vi "Upd Range.vi"(8 "error in (no error)":errorcluster, 11 "FC2901 in":refnum<class "FC2901.lvclass">) -> (0 "error out":errorcluster, 3 "FC2901 out":refnum<class "FC2901.lvclass">)   [LabVIEW 2021, in "FC2901.lvclass"]
uses:
  FC2901.lvclass
  FC2901.lvclass/FC2901.ctl
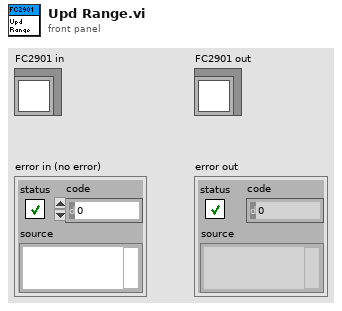
[diagram p1: front panel]
types:
  T1 = typedef "C100L.lvclass/GCF Data.ctl" = map{string, dbl}
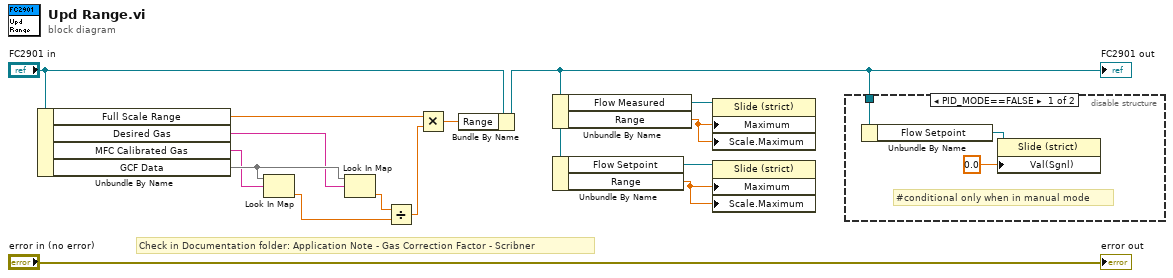
[diagram p0: block diagram]
diagram:
  # "Check in Documentation folder: Application Note - Gas Correction Factor - Scribner"
  n1 = Unbundle By Name("FC2901 in") -> ("Full Scale Range"=w10:dbl, "Desired Gas"=w11:string, "MFC Calibrated Gas"=w12:string, "GCF Data"=w13:T1)
  n2 = Look In Map(map=w13, key=w12) -> (value=w7:dbl)  [unwired: 1 in, 1 out]
  n3 = Look In Map(map=w13, key=w11) -> (value=w8:dbl)  [unwired: 1 in, 1 out]
  n4 = Divide(x=w8, y=w7) -> (x/y=w9:dbl)
  n5 = Multiply(x=w10, y=w9) -> (x*y=w2:dbl)
  n6 = Bundle By Name(cluster="FC2901 in", "Range"=w2) -> (w1:refnum<class "FC2901.lvclass">)
  "FC2901 out" <- w1
  n7 = Unbundle By Name(w1) -> ("Flow Measured"=w4:refnum<vi>, "Range"=w5:dbl)
  n8 = Unbundle By Name(w1) -> ("Flow Setpoint"=w3:refnum<vi>, "Range"=w6:dbl)
  n9 = property class="Slide (strict)"(reference=w4, "Maximum"=w5, "Scale.Maximum"=w5) -> ()  [unwired: 1 in, 2 out]
  n10 = property class="Slide (strict)"(reference=w3, "Maximum"=w6, "Scale.Maximum"=w6) -> ()  [unwired: 1 in, 2 out]
  n11 = disable-structure shown="PID_MODE==FALSE" {
    disable-tunnel: w1 -> [w17 _]
    frame condition #0 (active) {
      # "#conditional only when in manual mode"
      n12 = Unbundle By Name(w17) -> ("Flow Setpoint"=w18:refnum<vi>)
      n13 = property class="Slide (strict)"(reference=w18, "Val(Sgnl)"=0.0 ("Value (Signaling)")) -> ()  [unwired: 1 in, 2 out]
    }
    frame condition #1 {
    }
  }
  "error out" <- "error in (no error)"
